vi "Configure Waveform.vi"   [LabVIEW 2016, in "Agilent N6700 Series.lvlib"]
doc: "Configures a current or voltage waveform.\n\n<b>Note:</b>\n\nThis VI only applies to the N6705B DC Power Analyzer."
uses:
  <instrlib>/Agilent N6700 Series/Agilent N6700 Series.lvlib
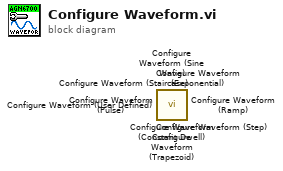
[diagram p0: block diagram]
diagram:
  n1 = call <instrlib>:"Configure Waveform (Constant Dwell).vi"() -> ()  [unwired: 14 in, 2 out]
  n2 = call <instrlib>:"Configure Waveform (Exponential).vi"() -> ()  [unwired: 14 in, 2 out]
  n3 = call <instrlib>:"Configure Waveform (Pulse).vi"() -> ()  [unwired: 14 in, 2 out]
  n4 = call <instrlib>:"Configure Waveform (Ramp).vi"() -> ()  [unwired: 14 in, 2 out]
  n5 = call <instrlib>:"Configure Waveform (Staircase).vi"() -> ()  [unwired: 14 in, 2 out]
  n6 = call <instrlib>:"Configure Waveform (Sine Wave).vi"() -> ()  [unwired: 14 in, 2 out]
  n7 = call <instrlib>:"Configure Waveform (Step).vi"() -> ()  [unwired: 14 in, 2 out]
  n8 = call <instrlib>:"Configure Waveform (Trapezoid).vi"() -> ()  [unwired: 14 in, 2 out]
  n9 = call <instrlib>:"Configure Waveform (User Defined).vi"() -> ()  [unwired: 14 in, 2 out]
